vi "MeasureLoop.vi"(8 "error in (no error)":errorcluster, 11 "Queue cluster":T1) -> ()   [LabVIEW 2017]
uses:
  QueueCluster.ctl
  EventQueueCluster.ctl
  EventMessage.ctl
  MeasureQueue.ctl
  MeasureMessage.ctl
  HardwareQueueCluster.ctl
  hardwareMessage.ctl
  GUIQueueCluster.ctl
  GUIMessage.ctl
  SaveQueueCluster.ctl
  SaveMessage.ctl
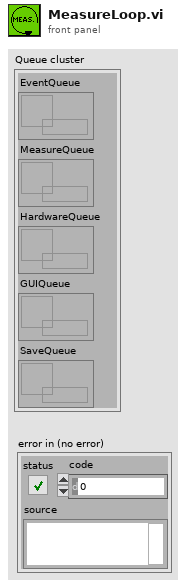
[diagram p1: front panel]
types:
  T1 = typedef "QueueCluster.ctl" = cluster{"EventQueue":refnum<queue>, "MeasureQueue":refnum<queue>, "HardwareQueue":refnum<queue>, "GUIQueue":refnum<queue>, "SaveQueue":refnum<queue>}
  T2 = typedef "MeasureQueue.ctl" = cluster{"NumericValue":dbl, "String":string, "MeasureMessage":T3}
  T3 = typedef "MeasureMessage.ctl" = enum16{"Init", "Measure", "Error", "Halt", "StartChannel", "StopChannel"}
  T4 = typedef "HardwareQueueCluster.ctl" = cluster{"HardwareMessage":T5, "NumericValue":dbl, "String":string}
  T5 = typedef "hardwareMessage.ctl" = enum16{"Init", "MeasureChannel", "CloseDevice", "Error", "Halt", "SetPhysChannel1", "SetPhysChannel2", "SetPhysChannel3"}
  T6 = typedef "GUIMessage.ctl" = enum16{"StopSave", "Channel1Value", "Channel2Value", "Channel3Value", "ErrorSource", "CleanError", "StartChannel1", "StartChannel2", "StartChannel3", "StopChannel1", "StopChannel2", "StopChannel3", "Halt"}
  T7 = typedef "GUIQueueCluster.ctl" = cluster{"GUIMessage":T6, "NumericValue":dbl, "String":string}
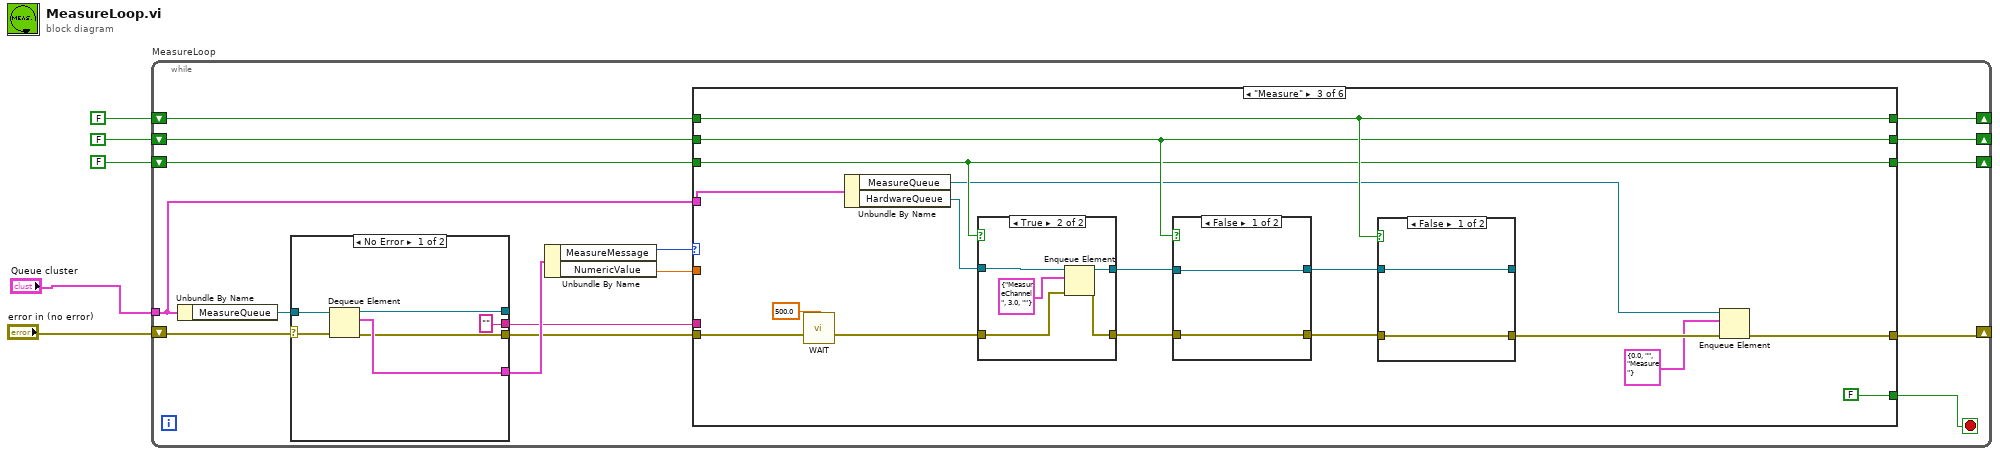
[diagram p0: block diagram]
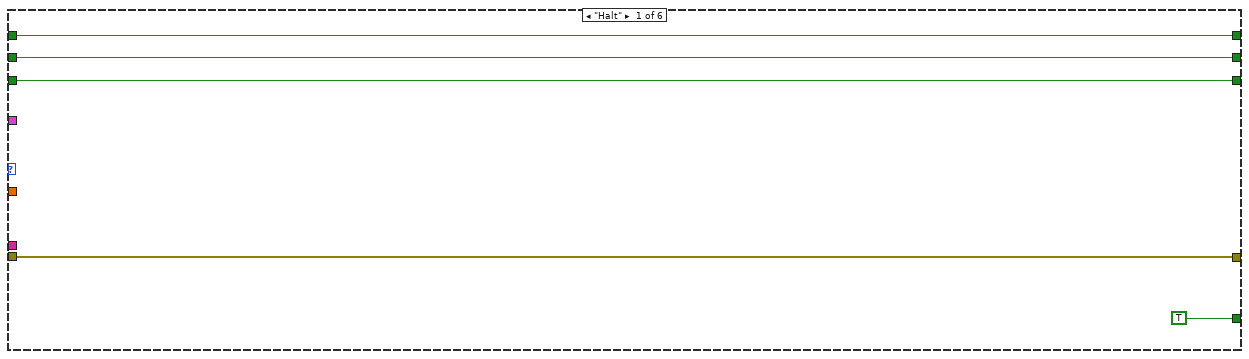
[diagram p2: hidden frame]
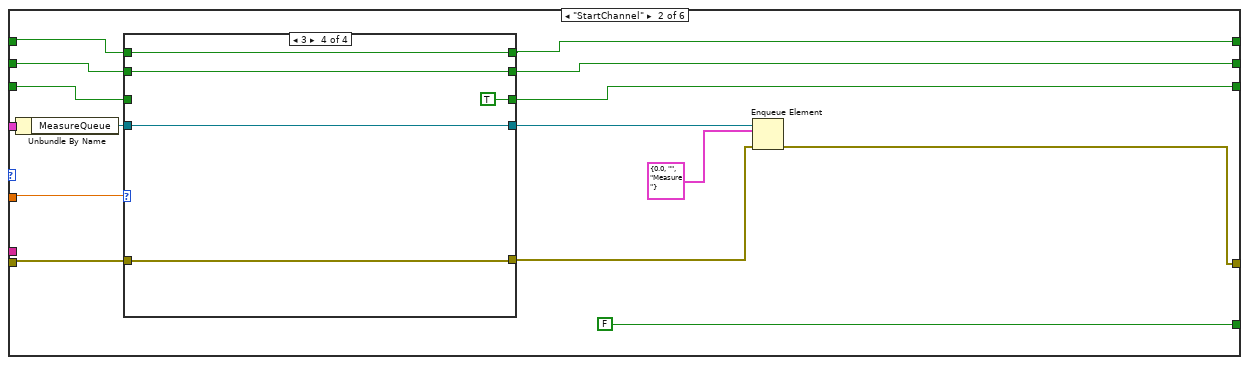
[diagram p3: hidden frame]
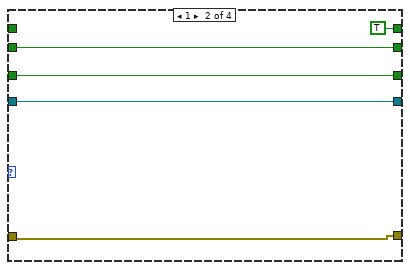
[diagram p5: hidden frame]
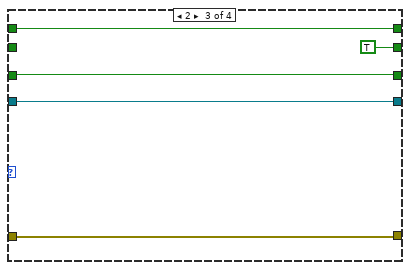
[diagram p6: hidden frame]
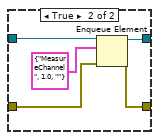
[diagram p7: hidden frame]
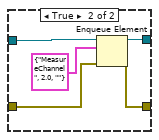
[diagram p8: hidden frame]
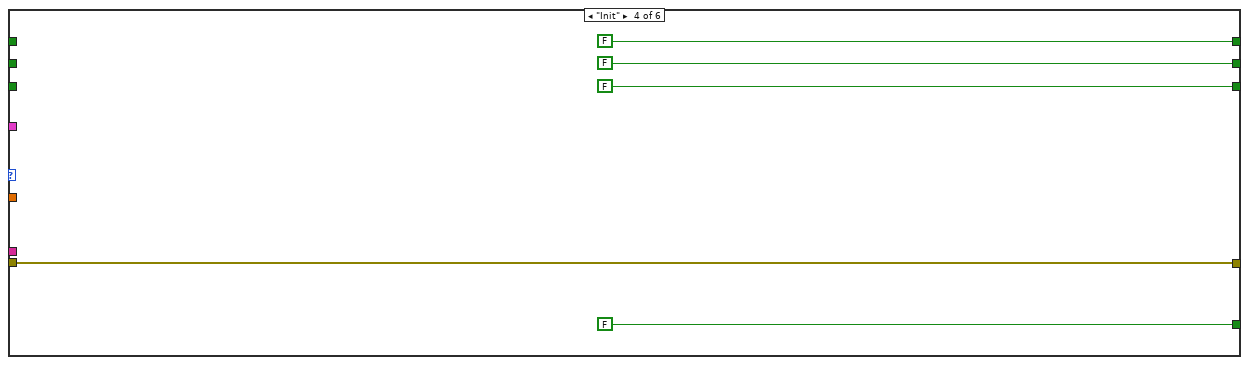
[diagram p10: hidden frame]
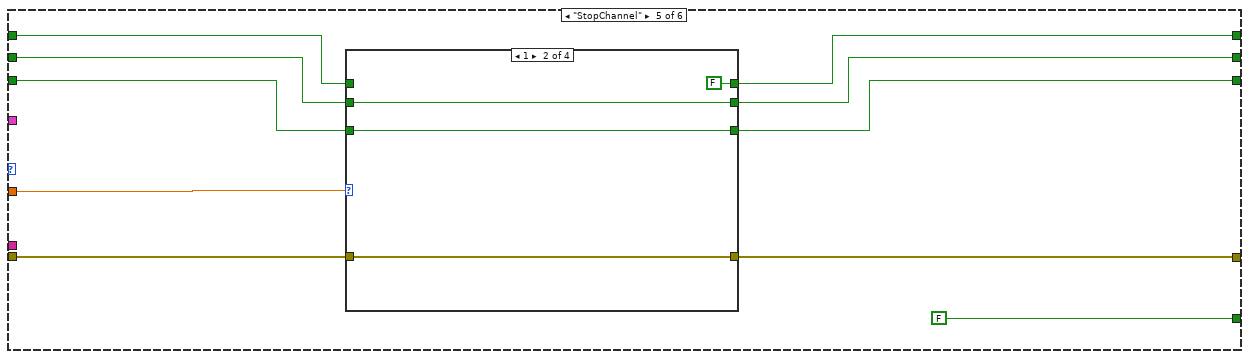
[diagram p11: hidden frame]
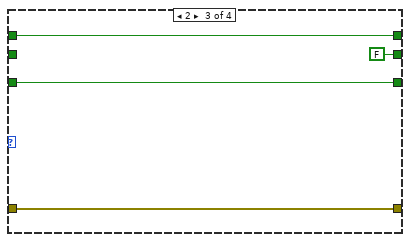
[diagram p13: hidden frame]
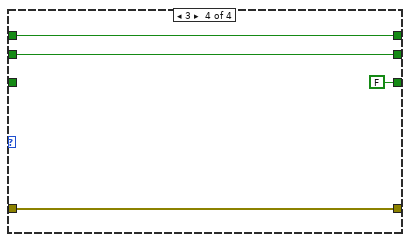
[diagram p14: hidden frame]
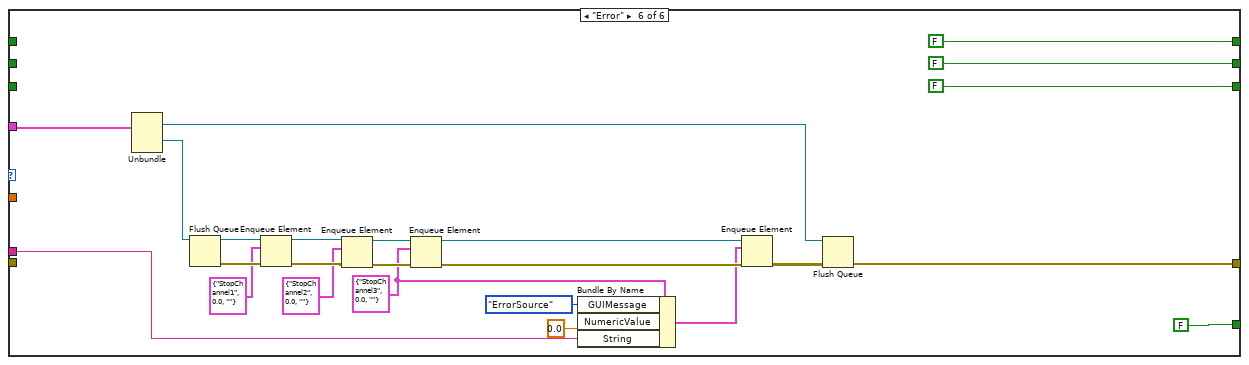
[diagram p15: hidden frame]
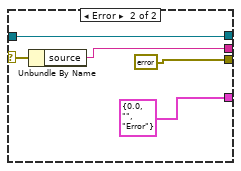
[diagram p16: hidden frame]
diagram:
  n1 = while "MeasureLoop" {
    tunnel: "Queue cluster" -> [w17]
    shift-right: [w8] -> _
    shift-left: "error in (no error)" -> [w16]
    shift-right: [w13] -> _
    shift-left: FALSE -> [w14]
    shift-right: [w11] -> _
    shift-left: FALSE -> [w12]
    shift-right: [w9] -> _
    shift-left: FALSE -> [w10]
    stop <- w18 stop-if-true
    n2 = Unbundle By Name(w17) -> ("MeasureQueue"=w21:refnum<queue>)
    n3 = case shown="No Error" w16 {
      selector: w16 -> [w160 w164]
      tunnel: w21 -> [w159 w165]
      tunnel: [w158 w165] -> _
      tunnel: [w157 T2 {"NumericValue"=0.0, "String"="", "MeasureMessage"=enum."Error"} ("MeasureQueue")] -> w20
      tunnel: [w156 errorcluster {"status"=FALSE, "code"=0, "source"=""} ("error out")] -> w15
      tunnel: ["" ("source") w163] -> w6
      frame No Error {
        n4 = Dequeue Element(queue=w159, error in (no error)=w160) -> (queue out=w158:refnum<queue>, element=w157:T2, error out=w156:errorcluster)  [unwired: 1 in, 1 out]
      }
      frame Error {
        n5 = Unbundle By Name(w164) -> ("source"=w163:string)
      }
    }
    n6 = Unbundle By Name(w20) -> ("MeasureMessage"=w19:T3, "NumericValue"=w7:dbl)
    n7 = case shown="\"Measure\"" w19 {
      tunnel: [TRUE FALSE FALSE FALSE FALSE FALSE] -> w18
      tunnel: w17 -> [_ w28 w78 _ _ w154]
      tunnel: w15 -> [w22 w34 w65 w104 w107 _]
      tunnel: [w25 w40 w71 FALSE w111 FALSE] -> w13
      tunnel: w14 -> [w25 w37 w71 _ w114 _]
      tunnel: [w24 w39 w70 FALSE w110 FALSE] -> w11
      tunnel: w12 -> [w24 w36 w70 _ w113 _]
      tunnel: w10 -> [w23 w35 w69 _ w112 _]
      tunnel: [w23 w38 w69 FALSE w109 FALSE] -> w9
      tunnel: [w22 w29 w67 w104 w106 w141] -> w8
      tunnel: w7 -> [_ w41 _ _ w108 _]
      tunnel: w6 -> [_ _ _ _ _ w139]
      frame "Halt" {
      }
      frame "StartChannel" {
        n8 = Unbundle By Name(w28) -> ("MeasureQueue"=w32:refnum<queue>)
        n9 = case shown="3" w41 {
          tunnel: [w46 TRUE w55 w61] -> w40
          tunnel: [w45 w51 TRUE w60] -> w39
          tunnel: [w44 w50 w56 TRUE] -> w38
          tunnel: w37 -> [w46 _ w55 w61]
          tunnel: w36 -> [w45 w51 _ w60]
          tunnel: w35 -> [w44 w50 w56 _]
          tunnel: w34 -> [w43 w48 w53 w58]
          tunnel: [w43 w48 w53 w58] -> w30
          tunnel: w32 -> [w42 w47 w52 w57]
          tunnel: [w42 w47 w52 w57] -> w31
          frame 0, Default {
          }
          frame 1 {
          }
          frame 2 {
          }
          frame 3 {
          }
        }
        n10 = Enqueue Element(queue=w31, element=T2 {"NumericValue"=0.0, "String"="", "MeasureMessage"=enum."Measure"}, error in (no error)=w30) -> (error out=w29:errorcluster)  [unwired: 1 in, 2 out]
      }
      frame "Measure" {
        n11 = call "WAIT.vi"("error in (no error)"=w65, "Time to wait"=500.0) -> ("error out"=w64:errorcluster)  [unwired: 13 in]
        n12 = Unbundle By Name(w78) -> ("MeasureQueue"=w66:refnum<queue>, "HardwareQueue"=w77:refnum<queue>)
        n13 = case shown="True" w69 {
          tunnel: w64 -> [w94 w99]
          tunnel: w77 -> [w93 w98]
          tunnel: [w94 w97] -> w75
          tunnel: [w93 w96] -> w76
          frame False {
          }
          frame True {
            n14 = Enqueue Element(queue=w98, element=T4 {"HardwareMessage"=enum."MeasureChannel", "NumericValue"=3.0, "String"=""}, error in (no error)=w99) -> (queue out=w96:refnum<queue>, error out=w97:errorcluster)  [unwired: 1 in, 1 out]
          }
        }
        n15 = case shown="False" w70 {
          tunnel: w75 -> [w87 w92]
          tunnel: w76 -> [w86 w91]
          tunnel: [w87 w90] -> w74
          tunnel: [w86 w89] -> w73
          frame False {
          }
          frame True {
            n16 = Enqueue Element(queue=w91, element=T4 {"HardwareMessage"=enum."MeasureChannel", "NumericValue"=2.0, "String"=""}, error in (no error)=w92) -> (queue out=w89:refnum<queue>, error out=w90:errorcluster)  [unwired: 1 in, 1 out]
          }
        }
        n17 = case shown="False" w71 {
          tunnel: w74 -> [w80 w85]
          tunnel: [w80 w84] -> w68
          tunnel: w73 -> [w79 w83]
          tunnel: [w79 w82] -> _
          frame False {
          }
          frame True {
            n18 = Enqueue Element(queue=w83, element=T4 {"HardwareMessage"=enum."MeasureChannel", "NumericValue"=1.0, "String"=""}, error in (no error)=w85) -> (queue out=w82:refnum<queue>, error out=w84:errorcluster)  [unwired: 1 in, 1 out]
          }
        }
        n19 = Enqueue Element(queue=w66, element=T2 {"NumericValue"=0.0, "String"="", "MeasureMessage"=enum."Measure"}, error in (no error)=w68) -> (error out=w67:errorcluster)  [unwired: 1 in, 2 out]
      }
      frame "Init" {
      }
      frame "StopChannel" {
        n20 = case shown="1" w108 {
          tunnel: [w118 FALSE w125 w130] -> w111
          tunnel: [w117 w122 FALSE w129] -> w110
          tunnel: [w116 w121 w126 FALSE] -> w109
          tunnel: w114 -> [w118 _ w125 w130]
          tunnel: w113 -> [w117 w122 _ w129]
          tunnel: w112 -> [w116 w121 w126 _]
          tunnel: w107 -> [w115 w119 w123 w127]
          tunnel: [w115 w119 w123 w127] -> w106
          frame 0, Default {
          }
          frame 1 {
          }
          frame 2 {
          }
          frame 3 {
          }
        }
      }
      frame "Error" {
        w133 = T7 {"GUIMessage"=enum."StopChannel3", "NumericValue"=0.0, "String"=""} ("element")
        n21 = Unbundle(w154) -> ("MeasureQueue"=w142:refnum<queue>, "GUIQueue"=w149:refnum<queue>)  [unwired: 3 out]
        n22 = Flush Queue(queue=w149) -> (queue out=w148:refnum<queue>, error out=w147:errorcluster)  [unwired: 1 in, 1 out]
        n23 = Enqueue Element(queue=w148, element=T7 {"GUIMessage"=enum."StopChannel1", "NumericValue"=0.0, "String"=""}, error in (no error)=w147) -> (queue out=w146:refnum<queue>, error out=w145:errorcluster)  [unwired: 1 in, 1 out]
        n24 = Enqueue Element(queue=w146, element=T7 {"GUIMessage"=enum."StopChannel2", "NumericValue"=0.0, "String"=""}, error in (no error)=w145) -> (queue out=w144:refnum<queue>, error out=w143:errorcluster)  [unwired: 1 in, 1 out]
        n25 = Enqueue Element(queue=w144, element=w133, error in (no error)=w143) -> (queue out=w140:refnum<queue>, error out=w138:errorcluster)  [unwired: 1 in, 1 out]
        n26 = Bundle By Name(cluster=w133, "GUIMessage"=GUIMessage."ErrorSource", "NumericValue"=0.0, "String"=w139) -> (w131:T7)
        n27 = Enqueue Element(queue=w140, element=w131, error in (no error)=w138) -> (error out=w137:errorcluster)  [unwired: 1 in, 2 out]
        n28 = Flush Queue(queue=w142, error in (no error)=w137) -> (error out=w141:errorcluster)  [unwired: 2 out]
      }
    }
  }
